vi "Read voltage range.vi"(8 "error in (no error)":errorcluster caption="에러 입력(에러 없음)", 11 "Waveform Obj 입력":refnum<class "Waveform Obj.lvclass">) -> (0 "error out":errorcluster caption="에러 출력", 2 "voltage range":dbl, 3 "Waveform Obj 출력":refnum<class "Waveform Obj.lvclass">)   [LabVIEW 2020, in "Waveform Obj.lvclass"]
uses:
  Waveform Obj.lvclass
  Waveform Obj.lvclass/Waveform Obj.ctl
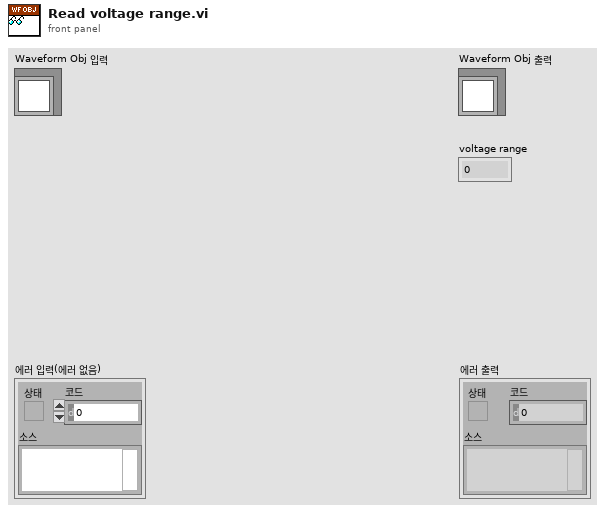
[diagram p1: front panel]
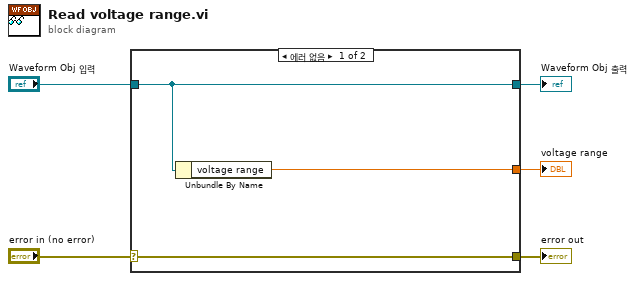
[diagram p0: block diagram]
diagram:
  n1 = case shown="에러 없음" "error in (no error)" {
    selector: "error in (no error)" -> [w8 w9]
    tunnel: [w8 w9] -> w4
    tunnel: [w7 w10] -> w2
    tunnel: "Waveform Obj 입력" -> [w7 w10]
    tunnel: [w6 _] -> w1
    frame No Error {
      n2 = Unbundle By Name(w7) -> ("voltage range"=w6:dbl)
    }
    frame Error {
    }
  }
  "error out" <- w4
  "Waveform Obj 출력" <- w2
  "voltage range" <- w1
